vi "Launch.vi"(8 "error in (no error)":errorcluster, 10 "Mediator":refnum<class "IMediator.lvclass">, 11 "IMediatorBusMonitor (Type)":refnum<class "IMediatorBusMonitor.lvclass">) -> (0 "error out":errorcluster, 1 "Bus Monitor Enqueuer":refnum<class "Message Enqueuer.lvclass">, 2 "Mediator Out":refnum<class "IMediator.lvclass">)   [LabVIEW 2015, in "IMediator.lvlib" / "IMediatorBusMonitor.lvclass"]
uses:
  IMediatorBusMonitor.lvclass
  IMediator/IMediator.lvclass
  <vilib>/ActorFramework/Message Enqueuer/Message Enqueuer.lvclass
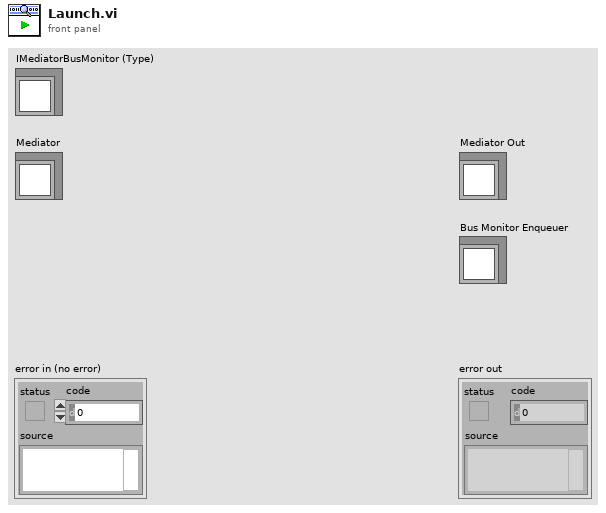
[diagram p1: front panel]
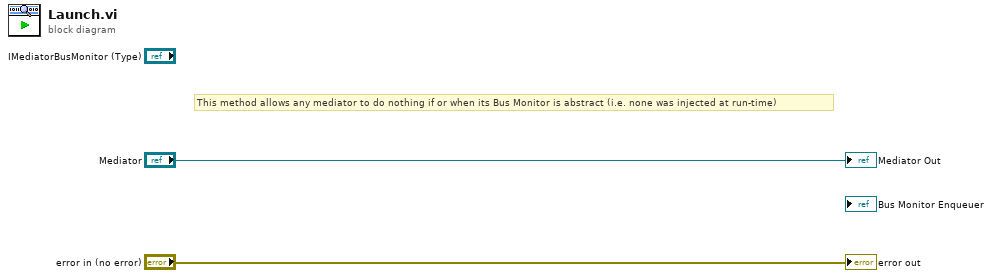
[diagram p0: block diagram]
diagram:
  # "This method allows any mediator to do nothing if or when its Bus Monitor is abstract (i.e. none was injected at run-time)"
  "error out" <- "error in (no error)"
  "Mediator Out" <- "Mediator"
